vi "Create Environment.vi"(7 "Environmental index":i32, 8 "error in (no error)":errorcluster, 10 "Environmental info":T1, 11 "XML Handler in":refnum<class "XML Handler.lvclass">) -> (0 "error out":errorcluster, 3 "XML Handler out":refnum<class "XML Handler.lvclass">)   [LabVIEW 2020, in "XML Handler.lvclass"]
doc: "Create the temperature element in the XML file"
uses:
  XML Handler.lvclass
  XML Handler.lvclass/XML Handler.ctl
  <vilib>/xml/Close Reference(Node).vi
  <resource>/objmgr/DOMUserDefRef.rc
  <vilib>/xml/NI_XML.lvlib
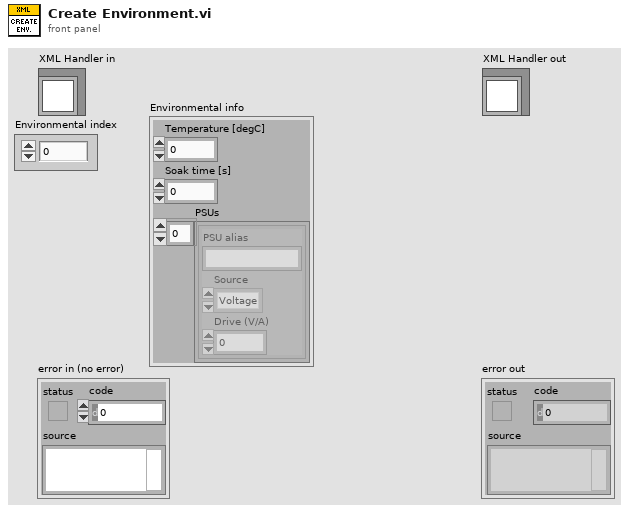
[diagram p1: front panel]
types:
  T1 = cluster{"Temperature [degC]":dbl, "Soak time [s]":dbl, "PSUs":cluster{"PSU alias":string, "Source":enum32{"Voltage", "Current"}, "Drive (V/A)":dbl}[]}
  T2 = cluster{"PSU alias":string, "Source":enum32{"Voltage", "Current"}, "Drive (V/A)":dbl}[]
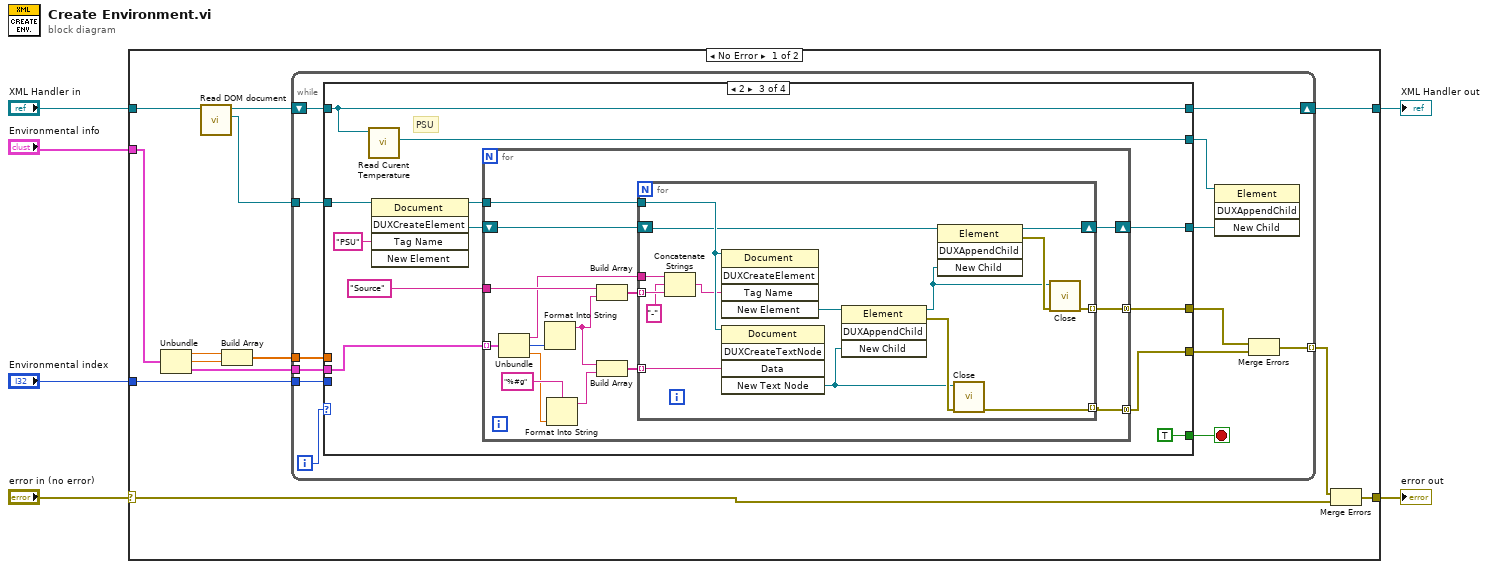
[diagram p0: block diagram]
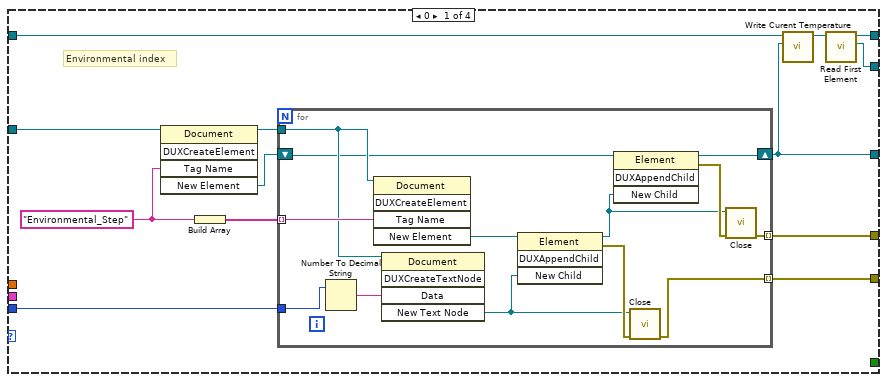
[diagram p2: hidden frame]
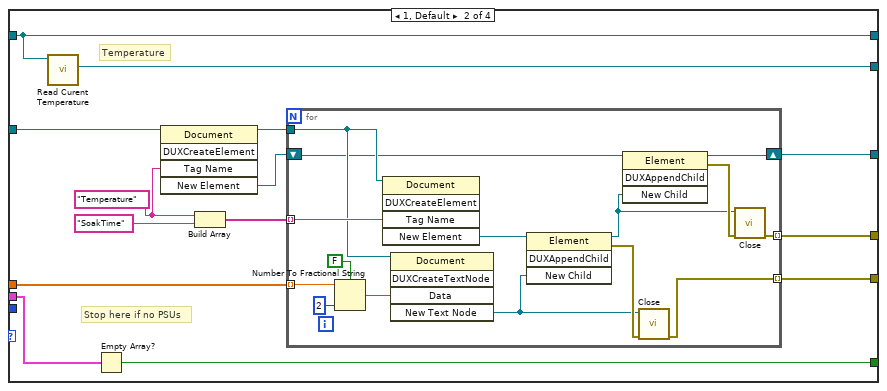
[diagram p3: hidden frame]
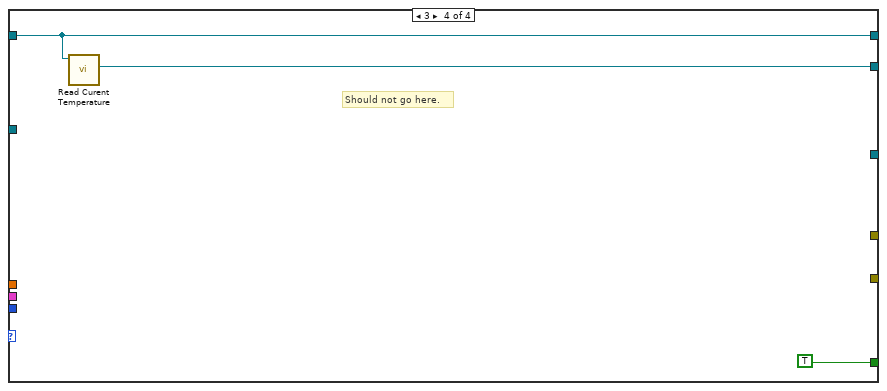
[diagram p4: hidden frame]
diagram:
  n1 = case shown="No Error" "error in (no error)" {
    selector: "error in (no error)" -> [w8 w134]
    tunnel: [w7 w134] -> w5
    tunnel: [w17 w133] -> w3
    tunnel: "XML Handler in" -> [w19 w133]
    tunnel: "Environmental info" -> [w16 _]
    tunnel: "Environmental index" -> [w10 _]
    frame No Error {
      n2 = Unbundle(w16) -> ("Temperature [degC]"=w15:dbl, "Soak time [s]"=w14:dbl, "PSUs"=w11:T2)
      n3 = call "Read DOM document.vi"("XML Handler in"=w19) -> ("DOM document"=w12:refnum<k20>, "XML Handler out"=w18:refnum<class "XML Handler.lvclass">)  [unwired: 9 in]
      n4 = Build Array(w15, w14) -> (w13:dbl[])
      n5 = while {
        tunnel: w13 -> [w32]
        tunnel: w12 -> [w31]
        shift-right: [w24] -> w17
        shift-left: w18 -> [w25]
        tunnel: w11 -> [w29]
        tunnel: w10 -> [w27]
        tunnel: [w20] -> w9 mode=indexing
        i -> [w30]
        stop <- w28 stop-if-true
        n6 = case shown="2" w30 {
          tunnel: [w38 w70 w98 _] -> w26
          tunnel: w32 -> [_ w66 _ _]
          tunnel: w31 -> [w40 w64 w97 _]
          tunnel: w29 -> [_ w62 w93 _]
          tunnel: [_ w61 TRUE TRUE] -> w28
          tunnel: w27 -> [w41 _ _ _]
          tunnel: [w36 w65 w91 w130] -> w24
          tunnel: w25 -> [w39 w65 w91 w130]
          tunnel: [w35 w63 w90 w131] -> w23
          tunnel: [w33 w59 w89 _] -> w22
          tunnel: [w34 w60 w88 _] -> w21
          frame 0 {
            w42 = "Environmental_Step" ("Tag Name")
            # "Environmental index"
            n7 = invoke class="Document" method="DUXCreateElement"(reference=w40, "Tag Name"=w42) -> (reference out=w43:refnum<k20>, "New Element"=w45:refnum<k20>)  [unwired: 3 in, 3 out]
            n8 = Build Array(w42) -> (w44:string[])
            n9 = for {
              tunnel: w44 -> [w58] mode=indexing
              tunnel: w43 -> [w57]
              shift-right: [w50] -> w38
              shift-left: w45 -> [w52]
              tunnel: w41 -> [w48]
              tunnel: [w47] -> w34 mode=indexing
              tunnel: [w46] -> w33 mode=indexing
              n10 = Number To Decimal String(number=w48) -> (decimal integer string=w56:string)  [unwired: 1 in]
              n11 = invoke class="Document" method="DUXCreateElement"(reference=w57, "Tag Name"=w58) -> ("New Element"=w55:refnum<k20>)  [unwired: 3 in, 4 out]
              n12 = invoke class="Document" method="DUXCreateTextNode"(reference=w57, "Data"=w56) -> ("New Text Node"=w53:refnum<k20>)  [unwired: 3 in, 4 out]
              n13 = invoke class="Element" method="DUXAppendChild"(reference=w55, "New Child"=w53) -> (reference out=w49:refnum<k20>, error out=w54:errorcluster)  [unwired: 2 in, 2 out]
              n14 = invoke class="Element" method="DUXAppendChild"(reference=w52, "New Child"=w49) -> (reference out=w50:refnum<k20>, error out=w51:errorcluster)  [unwired: 2 in, 2 out]
              n15 = call-poly <vilib>:"Close.vi"("error in (no error)"=w54, "node"=w53) -> ("error out"=w46:errorcluster)  [unwired: 7 in]
              n16 = call-poly <vilib>:"Close.vi"("error in (no error)"=w51, "node"=w49) -> ("error out"=w47:errorcluster)  [unwired: 7 in]
            }
            n17 = call "Write Curent Temperature.vi"("Curent Temperature"=w38, "XML Handler in"=w39) -> ("XML Handler out"=w37:refnum<class "XML Handler.lvclass">)  [unwired: 9 in]
            n18 = call "Read First Element.vi"("XML Handler in"=w37) -> ("First Element"=w35:refnum<k20>, "XML Handler out"=w36:refnum<class "XML Handler.lvclass">)  [unwired: 9 in]
          }
          frame 1, Default {
            w67 = "Temperature" ("Tag Name")
            # "Stop here if no PSUs"
            # "Temperature"
            n19 = call "Read Curent Temperature.vi"("XML Handler in"=w65) -> ("Curent Temperature"=w63:refnum<k20>)  [unwired: 9 in, 1 out]
            n20 = Empty Array?(array=w62) -> (empty?=w61:bool)
            n21 = invoke class="Document" method="DUXCreateElement"(reference=w64, "Tag Name"=w67) -> (reference out=w69:refnum<k20>, "New Element"=w72:refnum<k20>)  [unwired: 3 in, 3 out]
            n22 = Build Array(w67, "SoakTime" ("element")) -> (w71:string[])
            n23 = for {
              tunnel: w66 -> [w85] mode=indexing
              tunnel: w71 -> [w87] mode=indexing
              tunnel: w69 -> [w86]
              shift-right: [w76] -> w70
              shift-left: w72 -> [w78]
              tunnel: [w74] -> w60 mode=indexing
              tunnel: [w73] -> w59 mode=indexing
              n24 = Number To Fractional String(use system decimal point (T)=FALSE, number=w85, precision (6)=i16 2) -> (F-format string=w84:string)  [unwired: 1 in]
              n25 = invoke class="Document" method="DUXCreateElement"(reference=w86, "Tag Name"=w87) -> ("New Element"=w81:refnum<k20>)  [unwired: 3 in, 4 out]
              n26 = invoke class="Document" method="DUXCreateTextNode"(reference=w86, "Data"=w84) -> ("New Text Node"=w79:refnum<k20>)  [unwired: 3 in, 4 out]
              n27 = invoke class="Element" method="DUXAppendChild"(reference=w81, "New Child"=w79) -> (reference out=w75:refnum<k20>, error out=w80:errorcluster)  [unwired: 2 in, 2 out]
              n28 = invoke class="Element" method="DUXAppendChild"(reference=w78, "New Child"=w75) -> (reference out=w76:refnum<k20>, error out=w77:errorcluster)  [unwired: 2 in, 2 out]
              n29 = call-poly <vilib>:"Close.vi"("error in (no error)"=w80, "node"=w79) -> ("error out"=w73:errorcluster)  [unwired: 7 in]
              n30 = call-poly <vilib>:"Close.vi"("error in (no error)"=w77, "node"=w75) -> ("error out"=w74:errorcluster)  [unwired: 7 in]
            }
          }
          frame 2 {
            # "PSU"
            n31 = call "Read Curent Temperature.vi"("XML Handler in"=w91) -> ("Curent Temperature"=w90:refnum<k20>)  [unwired: 9 in, 1 out]
            n32 = invoke class="Document" method="DUXCreateElement"(reference=w97, "Tag Name"="PSU" ("element")) -> (reference out=w96:refnum<k20>, "New Element"=w99:refnum<k20>)  [unwired: 3 in, 3 out]
            n33 = for {
              tunnel: w96 -> [w112]
              shift-right: [w113] -> w98
              shift-left: w99 -> [w114]
              tunnel: w93 -> [w111] mode=indexing
              tunnel: "Source" ("element") -> [w110]
              tunnel: [w105] -> w89 mode=concatenating
              tunnel: [w104] -> w88 mode=concatenating
              n34 = Unbundle(w111) -> ("PSU alias"=w103:string, "Source"=w108:enum32{"Voltage", "Current"}, "Drive (V/A)"=w101:dbl)
              n35 = Format Into String(w108) -> (resulting string=w106:string)  [unwired: 3 in, 1 out]
              n36 = Format Into String(format string="%#g", w101) -> (resulting string=w100:string)  [unwired: 2 in, 1 out]
              n37 = Build Array(w110, w106) -> (w109:string[])
              n38 = Build Array(w106, w100) -> (w107:string[])
              n39 = for {
                tunnel: w109 -> [w118] mode=indexing
                tunnel: w112 -> [w129]
                shift-right: [w123] -> w113
                shift-left: w114 -> [w125]
                tunnel: w107 -> [w121] mode=indexing
                tunnel: [w120] -> w105 mode=indexing
                tunnel: [w119] -> w104 mode=indexing
                tunnel: w103 -> [w115]
                n40 = Concatenate Strings(w115, "-" ("string"), w118) -> (w117:string)
                n41 = invoke class="Document" method="DUXCreateElement"(reference=w129, "Tag Name"=w117) -> ("New Element"=w128:refnum<k20>)  [unwired: 3 in, 4 out]
                n42 = invoke class="Document" method="DUXCreateTextNode"(reference=w129, "Data"=w121) -> ("New Text Node"=w126:refnum<k20>)  [unwired: 3 in, 4 out]
                n43 = invoke class="Element" method="DUXAppendChild"(reference=w128, "New Child"=w126) -> (reference out=w122:refnum<k20>, error out=w127:errorcluster)  [unwired: 2 in, 2 out]
                n44 = invoke class="Element" method="DUXAppendChild"(reference=w125, "New Child"=w122) -> (reference out=w123:refnum<k20>, error out=w124:errorcluster)  [unwired: 2 in, 2 out]
                n45 = call-poly <vilib>:"Close.vi"("error in (no error)"=w127, "node"=w126) -> ("error out"=w120:errorcluster)  [unwired: 7 in]
                n46 = call-poly <vilib>:"Close.vi"("error in (no error)"=w124, "node"=w122) -> ("error out"=w119:errorcluster)  [unwired: 7 in]
              }
            }
          }
          frame 3 {
            # "Should not go here."
            n47 = call "Read Curent Temperature.vi"("XML Handler in"=w130) -> ("Curent Temperature"=w131:refnum<k20>)  [unwired: 9 in, 1 out]
          }
        }
        n48 = invoke class="Element" method="DUXAppendChild"(reference=w23, "New Child"=w26) -> ()  [unwired: 2 in, 4 out]
        n49 = Merge Errors(w21, w22) -> (w20:errorcluster)
      }
      n50 = Merge Errors(w9, w8) -> (w7:errorcluster)
    }
    frame Error {
    }
  }
  "error out" <- w5
  "XML Handler out" <- w3
